vi "WritePin.vi"(0 "NXP in":refnum<class "NXP.lvclass">, 5 "Port":dbl, 7 "Pin":dbl, 9 "Value":bool, 11 "error in (no error)":errorcluster) -> (4 "NXP out":refnum<class "NXP.lvclass">, 15 "error out":errorcluster)   [LabVIEW 2020, in "NXP.lvclass"]
uses:
  NXP.lvclass
  Abstract/Serial Device/Serial Device.lvclass
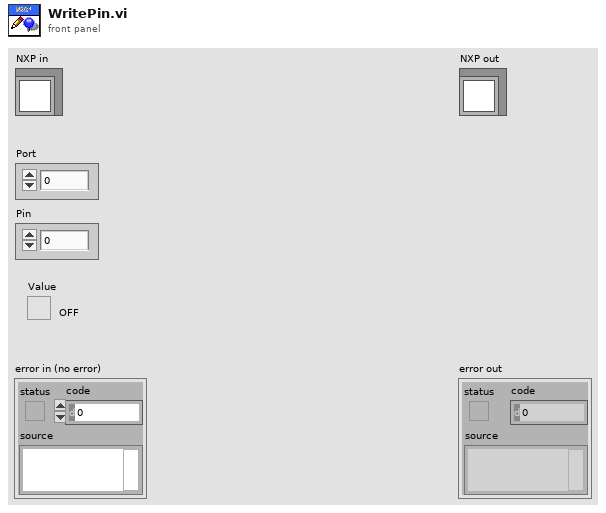
[diagram p1: front panel]
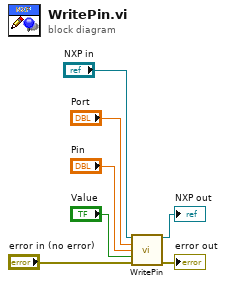
[diagram p0: block diagram]
diagram:
  n1 = call-parent "WritePin.vi"("Serial Device in"="NXP in", "Port"="Port", "Pin"="Pin", "Value"="Value", "error in (no error)"="error in (no error)") -> ("Serial Device out"=→"NXP out":refnum<class "NXP.lvclass">, "error out"=→"error out":errorcluster)  [unwired: 9 in]
